vi "Config file path--constant.vi"() -> (3 "Path":path)   [LabVIEW 2020, in "UI.lvlib"]
uses:
  UI.lvlib
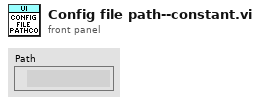
[diagram p1: front panel]
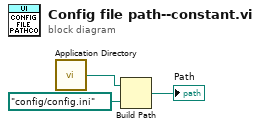
[diagram p0: block diagram]
diagram:
  n1 = call <vilib>:"Application Directory.vi"() -> ("Application Directory"=w3:path)
  n2 = Build Path(base path=w3, name or relative path=path "config/config.ini") -> (appended path=→"Path":path)
